vi "INS Decode (SubVI).vi"(10 "read buffer":string) -> (2 "Data out":dbl[](array[numeric]))   [LabVIEW 2021]
panel:
  out "Valid Data":string
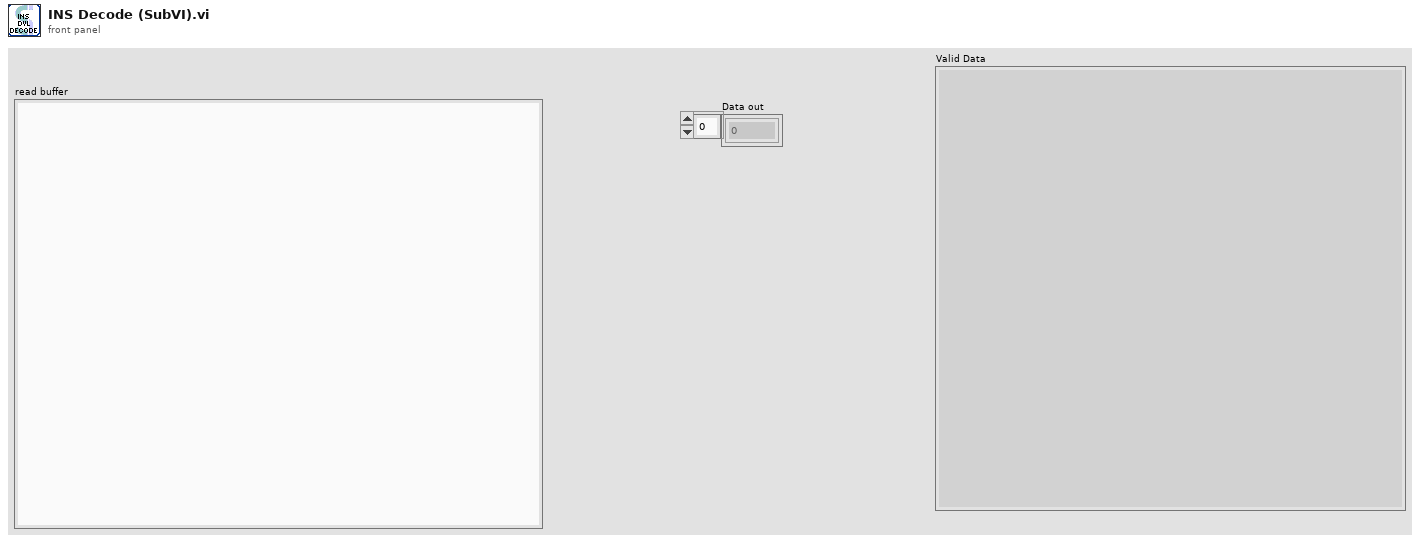
[diagram p1: front panel]
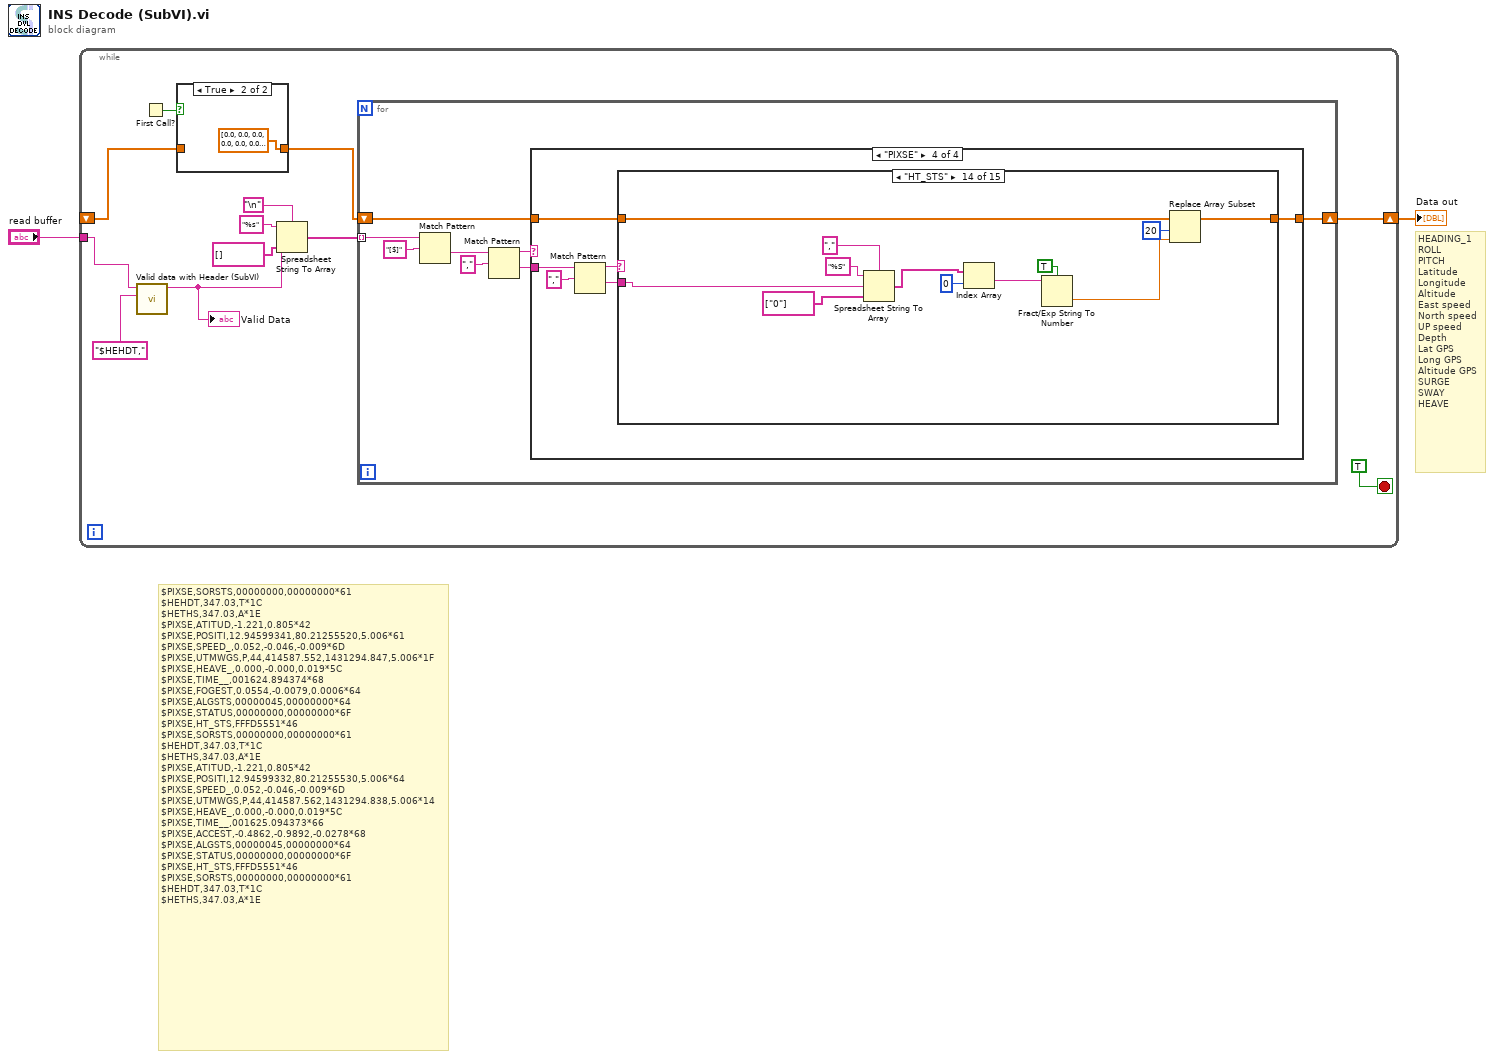
[diagram p0: block diagram]
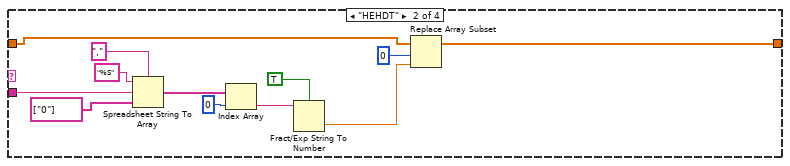
[diagram p4: hidden frame]
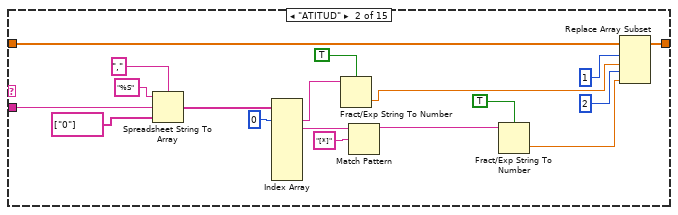
[diagram p7: hidden frame]
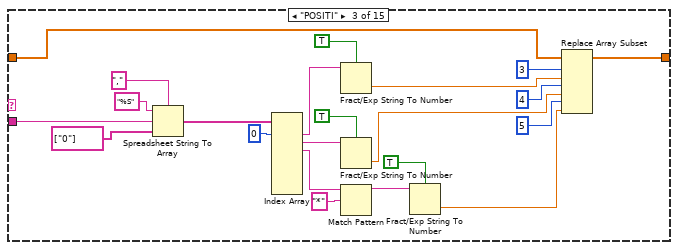
[diagram p8: hidden frame]
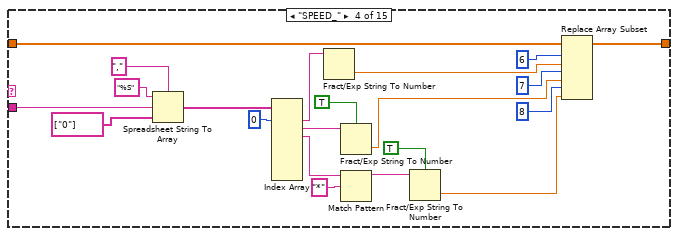
[diagram p9: hidden frame]
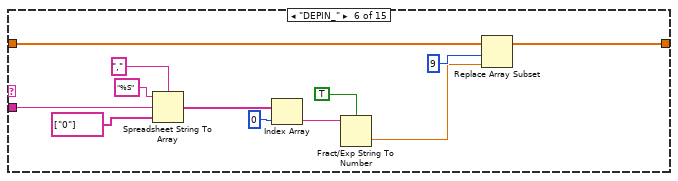
[diagram p11: hidden frame]
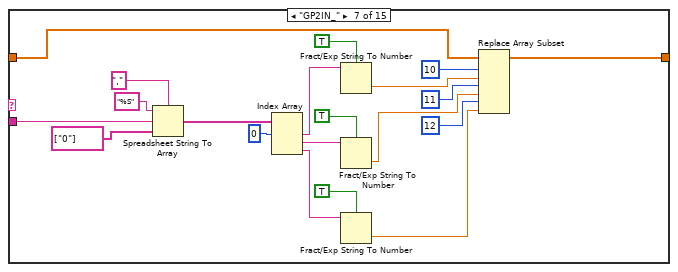
[diagram p12: hidden frame]
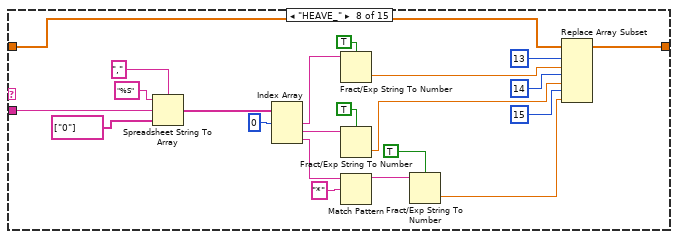
[diagram p13: hidden frame]
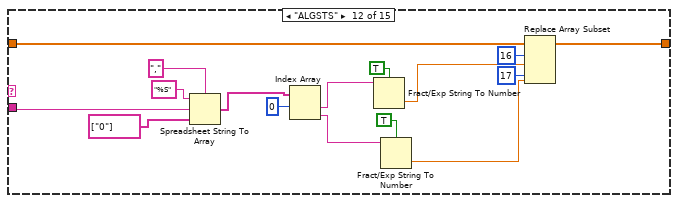
[diagram p17: hidden frame]
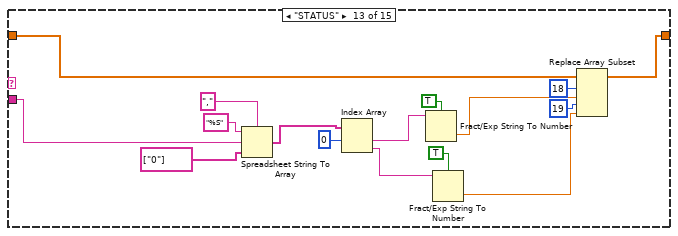
[diagram p18: hidden frame]
diagram:
  # "$PIXSE,SORSTS,00000000,00000000*61\n$HEHDT,347.03,T*1C\n$HETHS,347.03,A*1E\n$PIXSE,ATITUD,-1.221,0.805*42\n$PIXSE,POSITI,12.94599341,80.21255520,5.006*61\n$PIXSE,SPEED_,0.052,-0.046,-0.009*6D\n$PIXSE,UTMWGS,P,44,414587.552,1431294.847,5.006*1F\n$PIXSE,HEAVE_,0.000,-0.000,0.019*5C\n$PIXSE,TIME__,001624.894374*68\n$PIXSE,FOGEST,0.0554,-0.0079,0.0006*64\n$PIXSE,ALGSTS,00000045,00000000*64\n$PIXSE,STATUS,00000000,00000000*6F\n$PIXSE,HT_STS,FFFD5551*46\n$PIXSE,SORSTS,00000000,00000000*61\n$HEHDT,347.03,T*1C\n$HETHS,347.03,A*1E\n$PIXSE,ATITUD,-1.221,0.805*42\n$PIXSE,POSITI,12.94599332,80.21255530,5.006*64\n$PIXSE,SPEED_,0.052,-0.046,-0.009*6D\n$PIXSE,UTMWGS,P,44,414587.562,1431294.838,5.006*14\n$PIXSE,HEAVE_,0.000,-0.000,0.019*5C\n$PIXSE,TIME__,001625.094373*66\n$PIXSE,ACCEST,-0.4862,-0.9892,-0.0278*68\n$PIXSE,ALGSTS,00000045,00000000*64\n$PIXSE,STATUS,00000000,00000000*6F\n$PIXSE,HT_STS,FFFD5551*46\n$PIXSE,SORSTS,00000000,00000000*61\n$HEHDT,347.03,T*1C\n$HETHS,347.03,A*1E"
  # "HEADING_1\nROLL\nPITCH\nLatitude\nLongitude\nAltitude\nEast speed\nNorth speed\nUP speed\nDepth\nLat GPS\nLong GPS\nAltitude GPS\nSURGE\nSWAY\nHEAVE"
  n1 = while {
    tunnel: "read buffer" -> [w4]
    shift-right: [w10] -> w2
    shift-left: _ -> [w7]
    stop <- TRUE stop-if-true
    n2 = call "Valid data with Header (SubVI).vi"("Header"="$HEHDT," ("regular expression"), "Input data"=w4) -> ("Valid Data"=w3:string)  [unwired: 9 in]
    "Valid Data" <- w3
    n3 = First Call?() -> (First Call?: T/F=w9:bool)
    n4 = case shown="True" w9 {
      tunnel: [w15 dbl[] [0.0, 0.0, 0.0, 0.0, 0.0, 0.0, 0.0, 0.0, 0.0, 0.0, 0.0, 0.0, 0.0, 0.0, 0.0, 0.0, 0.0, 0.0, 0.0, 0.0, 0.0]] -> w8
      tunnel: w7 -> [w15 _]
      frame False {
      }
      frame True {
      }
    }
    n5 = Spreadsheet String To Array(delimiter (Tab)="\n", format string="%s", spreadsheet string=w3, array type (2D Dbl)=string[] []) -> (array=w11:string[])
    n6 = for {
      tunnel: w11 -> [w19] mode=indexing
      shift-right: [w18] -> w10
      shift-left: w8 -> [w17]
      n7 = Match Pattern(string=w19, regular expression="[$]") -> (after substring=w23:string)  [unwired: 1 in, 3 out]
      n8 = Match Pattern(string=w23, regular expression=",") -> (before substring=w21:string, after substring=w20:string)  [unwired: 1 in, 2 out]
      n9 = case shown="\"PIXSE\"" w21 {
        tunnel: w20 -> [_ w34 _ w44]
        tunnel: w17 -> [w25 w29 w38 w40]
        tunnel: [w25 w28 w38 w39] -> w18
        frame "False", Default {
        }
        frame "HEHDT" {
          n10 = Spreadsheet String To Array(delimiter (Tab)=",", format string="%S", spreadsheet string=w34, array type (2D Dbl)=string[] ["0"]) -> (array=w32:string[])
          n11 = Index Array(array=w32, index=0) -> (element=w30:string)
          n12 = Fract/Exp String To Number(use system decimal point (T)=TRUE, string=w30) -> (number=w26:dbl)  [unwired: 2 in, 1 out]
          n13 = Replace Array Subset(array=w29, new element=w26, index=0) -> (w28:dbl[])
        }
        frame "HETHS" {
        }
        frame "PIXSE" {
          n14 = Match Pattern(string=w44, regular expression=",") -> (before substring=w42:string, after substring=w41:string)  [unwired: 1 in, 2 out]
          n15 = case shown="\"HT_STS\"" w42 {
            tunnel: w41 -> [_ w60 w82 w103 _ w112 w132 w161 _ _ _ w177 w191 w203 _]
            tunnel: w40 -> [w45 w51 w70 w92 w107 w110 w127 w146 w162 w163 w164 w170 w193 w201 w209]
            tunnel: [w45 w50 w71 w93 w107 w111 w126 w147 w162 w163 w164 w169 w192 w197 w209] -> w39
            frame "False", Default {
            }
            frame "ATITUD" {
              n16 = Spreadsheet String To Array(delimiter (Tab)=",", format string="%S", spreadsheet string=w60, array type (2D Dbl)=string[] ["0"]) -> (array=w59:string[])
              n17 = Index Array(array=w59, index #1=0 ("index")) -> (element #1=w55:string, element #2=w56:string)  [unwired: 7 in, 6 out]
              n18 = Fract/Exp String To Number(use system decimal point (T)=TRUE, string=w55) -> (number=w48:dbl)  [unwired: 2 in, 1 out]
              n19 = Match Pattern(string=w56, regular expression="[*]") -> (before substring=w53:string)  [unwired: 1 in, 3 out]
              n20 = Fract/Exp String To Number(use system decimal point (T)=TRUE, string=w53) -> (number=w47:dbl)  [unwired: 2 in, 1 out]
              n21 = Replace Array Subset(array=w51, new element #1=w48, index #1=1 ("index"), new element #2=w47, index #2=2 ("index")) -> (w50:dbl[])
            }
            frame "POSITI" {
              n22 = Spreadsheet String To Array(delimiter (Tab)=",", format string="%S", spreadsheet string=w82, array type (2D Dbl)=string[] ["0"]) -> (array=w79:string[])
              n23 = Index Array(array=w79, index #1=0 ("index")) -> (element #1=w81:string, element #2=w72:string, element #3=w74:string)  [unwired: 7 in, 5 out]
              n24 = Fract/Exp String To Number(use system decimal point (T)=TRUE, string=w81) -> (number=w68:dbl)  [unwired: 2 in, 1 out]
              n25 = Fract/Exp String To Number(use system decimal point (T)=TRUE, string=w72) -> (number=w67:dbl)  [unwired: 2 in, 1 out]
              n26 = Match Pattern(string=w74, regular expression="*") -> (before substring=w76:string)  [unwired: 1 in, 3 out]
              n27 = Fract/Exp String To Number(use system decimal point (T)=TRUE, string=w76) -> (number=w66:dbl)  [unwired: 2 in, 1 out]
              n28 = Replace Array Subset(array=w70, new element #1=w68, index #1=3 ("index"), new element #2=w67, index #2=4 ("index"), new element #3=w66, index #3=5 ("index")) -> (w71:dbl[])
            }
            frame "SPEED_" {
              n29 = Spreadsheet String To Array(delimiter (Tab)=",", format string="%S", spreadsheet string=w103, array type (2D Dbl)=string[] ["0"]) -> (array=w94:string[])
              n30 = Index Array(array=w94, index #1=0 ("index")) -> (element #1=w102:string, element #2=w95:string, element #3=w97:string)  [unwired: 7 in, 5 out]
              n31 = Fract/Exp String To Number(string=w102) -> (number=w90:dbl)  [unwired: 3 in, 1 out]
              n32 = Fract/Exp String To Number(use system decimal point (T)=TRUE, string=w95) -> (number=w89:dbl)  [unwired: 2 in, 1 out]
              n33 = Match Pattern(string=w97, regular expression="*") -> (before substring=w99:string)  [unwired: 1 in, 3 out]
              n34 = Fract/Exp String To Number(use system decimal point (T)=TRUE, string=w99) -> (number=w88:dbl)  [unwired: 2 in, 1 out]
              n35 = Replace Array Subset(array=w92, new element #1=w90, index #1=6 ("index"), new element #2=w89, index #2=7 ("index"), new element #3=w88, index #3=8 ("index")) -> (w93:dbl[])
            }
            frame "UTMWGS" {
            }
            frame "DEPIN_" {
              n36 = Spreadsheet String To Array(delimiter (Tab)=",", format string="%S", spreadsheet string=w112, array type (2D Dbl)=string[] ["0"]) -> (array=w116:string[])
              n37 = Index Array(array=w116, index=0) -> (element=w114:string)
              n38 = Fract/Exp String To Number(use system decimal point (T)=TRUE, string=w114) -> (number=w108:dbl)  [unwired: 2 in, 1 out]
              n39 = Replace Array Subset(array=w110, new element=w108, index=9) -> (w111:dbl[])
            }
            frame "GP2IN_" {
              n40 = Spreadsheet String To Array(delimiter (Tab)=",", format string="%S", spreadsheet string=w132, array type (2D Dbl)=string[] ["0"]) -> (array=w134:string[])
              n41 = Index Array(array=w134, index #1=0 ("index")) -> (element #1=w129:string, element #2=w128:string, element #3=w133:string)  [unwired: 2 in]
              n42 = Fract/Exp String To Number(use system decimal point (T)=TRUE, string=w129) -> (number=w122:dbl)  [unwired: 2 in, 1 out]
              n43 = Fract/Exp String To Number(use system decimal point (T)=TRUE, string=w128) -> (number=w121:dbl)  [unwired: 2 in, 1 out]
              n44 = Fract/Exp String To Number(use system decimal point (T)=TRUE, string=w133) -> (number=w120:dbl)  [unwired: 2 in, 1 out]
              n45 = Replace Array Subset(array=w127, new element #1=w122, index #1=10 ("index"), new element #2=w121, index #2=11 ("index"), new element #3=w120, index #3=12 ("index")) -> (w126:dbl[])
            }
            frame "HEAVE_" {
              n46 = Spreadsheet String To Array(delimiter (Tab)=",", format string="%S", spreadsheet string=w161, array type (2D Dbl)=string[] ["0"]) -> (array=w149:string[])
              n47 = Index Array(array=w149, index #1=0 ("index")) -> (element #1=w154:string, element #2=w157:string, element #3=w156:string)  [unwired: 2 in]
              n48 = Fract/Exp String To Number(use system decimal point (T)=TRUE, string=w154) -> (number=w144:dbl)  [unwired: 2 in, 1 out]
              n49 = Fract/Exp String To Number(use system decimal point (T)=TRUE, string=w157) -> (number=w143:dbl)  [unwired: 2 in, 1 out]
              n50 = Match Pattern(string=w156, regular expression="*") -> (before substring=w155:string)  [unwired: 1 in, 3 out]
              n51 = Fract/Exp String To Number(use system decimal point (T)=TRUE, string=w155) -> (number=w142:dbl)  [unwired: 2 in, 1 out]
              n52 = Replace Array Subset(array=w146, new element #1=w144, index #1=13 ("index"), new element #2=w143, index #2=14 ("index"), new element #3=w142, index #3=15 ("index")) -> (w147:dbl[])
            }
            frame "STDHRP" {
            }
            frame "STDPOS" {
            }
            frame "STDSPD" {
            }
            frame "ALGSTS" {
              n53 = Spreadsheet String To Array(delimiter (Tab)=",", format string="%S", spreadsheet string=w177, array type (2D Dbl)=string[] ["0"]) -> (array=w173:string[])
              n54 = Index Array(array=w173, index #1=0 ("index")) -> (element #1=w172:string, element #2=w171:string)  [unwired: 1 in]
              n55 = Fract/Exp String To Number(use system decimal point (T)=TRUE, string=w172) -> (number=w168:dbl)  [unwired: 2 in, 1 out]
              n56 = Fract/Exp String To Number(use system decimal point (T)=TRUE, string=w171) -> (number=w167:dbl)  [unwired: 2 in, 1 out]
              n57 = Replace Array Subset(array=w170, new element #1=w168, index #1=16 ("index"), new element #2=w167, index #2=17 ("index")) -> (w169:dbl[])
            }
            frame "STATUS" {
              n58 = Spreadsheet String To Array(delimiter (Tab)=",", format string="%S", spreadsheet string=w191, array type (2D Dbl)=string[] ["0"]) -> (array=w194:string[])
              n59 = Index Array(array=w194, index #1=0 ("index")) -> (element #1=w184:string, element #2=w183:string)  [unwired: 1 in]
              n60 = Fract/Exp String To Number(use system decimal point (T)=TRUE, string=w184) -> (number=w195:dbl)  [unwired: 2 in, 1 out]
              n61 = Fract/Exp String To Number(use system decimal point (T)=TRUE, string=w183) -> (number=w196:dbl)  [unwired: 2 in, 1 out]
              n62 = Replace Array Subset(array=w193, new element #1=w195, index #1=18 ("index"), new element #2=w196, index #2=19 ("index")) -> (w192:dbl[])
            }
            frame "HT_STS" {
              n63 = Spreadsheet String To Array(delimiter (Tab)=",", format string="%S", spreadsheet string=w203, array type (2D Dbl)=string[] ["0"]) -> (array=w208:string[])
              n64 = Index Array(array=w208, index=0) -> (element=w199:string)
              n65 = Fract/Exp String To Number(use system decimal point (T)=TRUE, string=w199) -> (number=w198:dbl)  [unwired: 2 in, 1 out]
              n66 = Replace Array Subset(array=w201, new element=w198, index=20) -> (w197:dbl[])
            }
            frame "TIME__" {
            }
          }
        }
      }
    }
  }
  "Data out" <- w2
